vi "Voltage - Continuous Output.vi"(0 "Physical Channel(s)":tag="Dev1/ao0", 1 "Output Array":T2(array[cluster])=[{"Waveform Type"=0, "Amplitude"=1.0, "Frequency"=10.0}] {"Frequency" format="%0.2p"; "Amplitude" format="%0.2p"; "Waveform Type" items=["Sine Wave", "Triangle Wave", "Square Wave", "Sawtooth Wave"]}, 4 "Sample Rate":dbl=100000.0, 5 "Stop":bool, 7 "error in":errorcluster) -> (20 "Waveform Graph":waveform(dbl)[](graph)=[{"t0"=timestamp(0 s since 1904-01-01), "dt"=0.001, "Y"=[]}], 27 "error out":errorcluster)   [LabVIEW 2020]
uses:
  <vilib>/Utility/error.llb/DialogType.ctl
  <vilib>/DAQmx/write.llb/DAQmx Write (Analog 1D Wfm NChan NSamp).vi
  <vilib>/DAQmx/create/channels.llb/DAQmx Create Channel (AO-Voltage-Basic).vi
  <vilib>/DAQmx/configure/timing.llb/DAQmx Timing (Sample Clock).vi
  <vilib>/DAQmx/configure/trigger.llb/DAQmx Start Trigger (Digital Edge).vi
  <vilib>/DAQmx/configure/trigger.llb/DAQmx Start Trigger (Time).vi
  <vilib>/DAQmx/configure/trigger.llb/DAQmx Start Trigger (Analog Edge).vi
  <vilib>/DAQmx/miscellaneous.llb/DAQmx Fill In Error Info.vi
  <resource>/objmgr/daqmx.rc
  <vilib>/measure/NI_MABase.lvlib
panel:
  in  "Trigger Type":T1(tab)
  in  "Digital Start Trigger Edge":i32(ring)=10280 caption="Edge" items=["Rising"=10280, "Falling"=10171]
  in  "Digital Start Trigger Source":tag="/Dev1/PFI0" caption="Source"
  in  "Digital Pause Trigger Pause When":i32(ring)=10192 caption="Pause When" items=["High"=10192, "Low"=10214]
  in  "Digital Pause Trigger Source":tag="/Dev1/PFI0" caption="Source"
  in  "Analog Start Trigger Level":dbl caption="Level" format="%0.2f"
  in  "Analog Start Trigger Hysteresis":dbl caption="Hysteresis" format="%.2f"
  in  "Analog Start Trigger Slope":i32(ring)=10280 caption="Slope" items=["Rising"=10280, "Falling"=10171]
  in  "Analog Start Trigger Source":string="APFI0" caption="Source"
  in  "Analog Pause Trigger Source":string="APFI0" caption="Source"
  in  "Analog Pause Trigger Pause When":i32(ring)=10093 caption="Pause When" items=["Above Level"=10093, "Below Level"=10107]
  in  "Analog Pause Trigger Level":dbl caption="Level" format="%.2f"
  in  "When":timestamp
  in  "Select Time\nManually":bool
  in  "Number of Samples":i32=10000
  in  "Sample Clock Source":tag="OnboardClock"
  in  "Max Voltage":dbl=5.0
  in  "Min Voltage":dbl=-5.0
  out "Actual Sample Rate":dbl=1000.0 format="%0.2f"
  # "Channel Settings"
  # "Output"
  # "Timing and\nBuffer Settings"
  # "Waveform Settings"
  # "Trigger Settings"
  # "The number of elements in the waveform array must equal the number of channels in the task."
  # "To enable triggers, select a tab above, and configure the settings.\n\nNot all hardware supports all trigger types. Refer to your device documentation for more information."
  # "This trigger type is not supported in output tasks. \n\nRefer to your device documentation for more information on which triggers are supported."
  # "This trigger type is not supported in output tasks. \n\nRefer to your device documentation for more information on which triggers are supported."
  # "If time is not manually set, task will begin after 10 seconds"
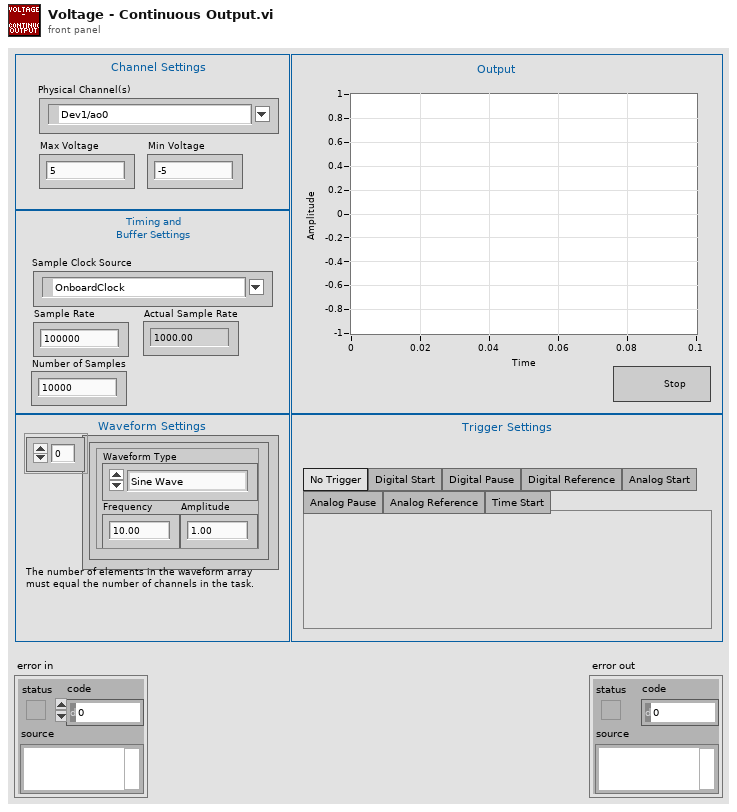
[diagram p1: front panel]
types:
  T1 = enum32{"No Trigger", "Digital Start", "Digital Pause", "Digital Reference", "Analog Start", "Analog Pause", "Analog Reference", "Time Start"}
  T2 = cluster{"Waveform Type":u16, "Amplitude":dbl, "Frequency":dbl}[]
  T3 = typedef "DialogType.ctl" = u16
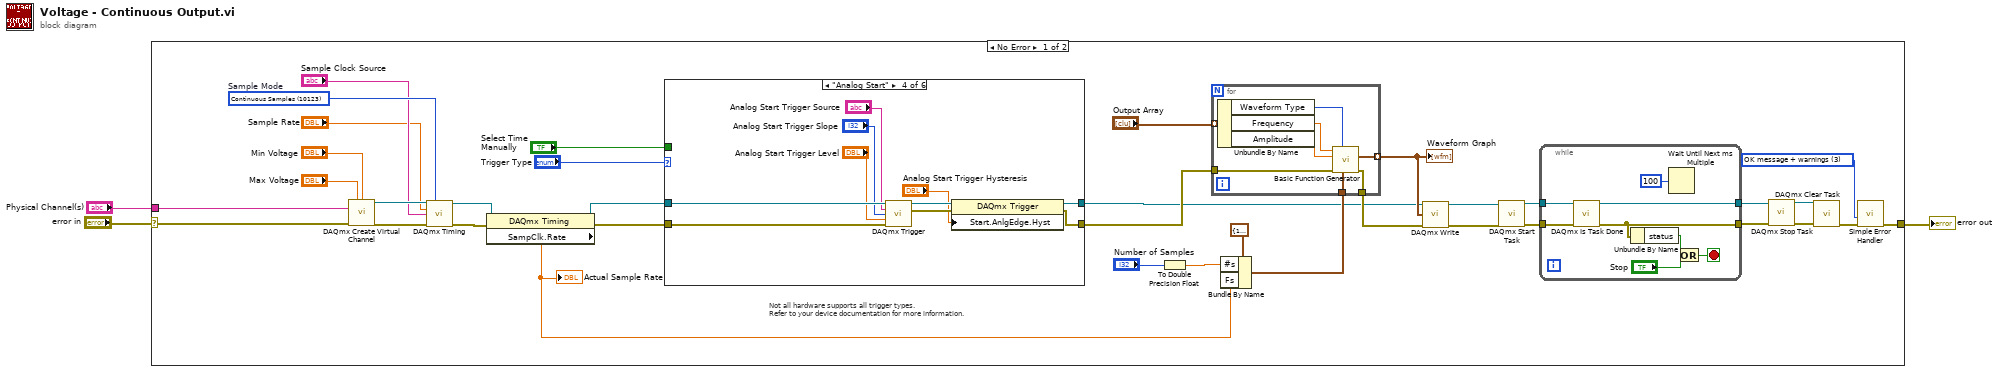
[diagram p0: block diagram]
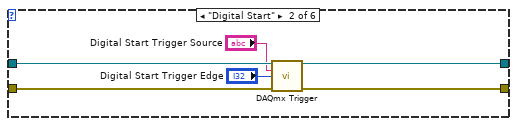
[diagram p3: hidden frame]
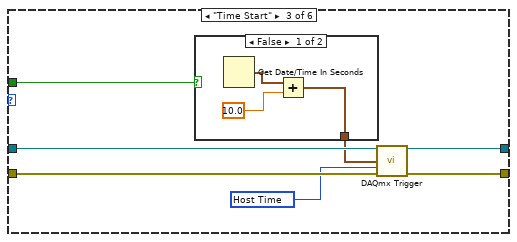
[diagram p4: hidden frame]
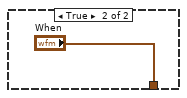
[diagram p5: hidden frame]
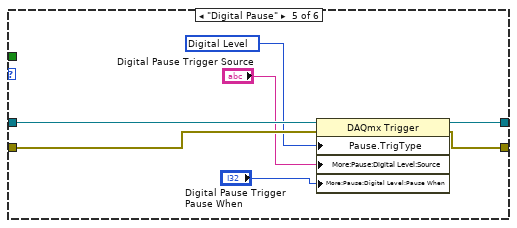
[diagram p6: hidden frame]
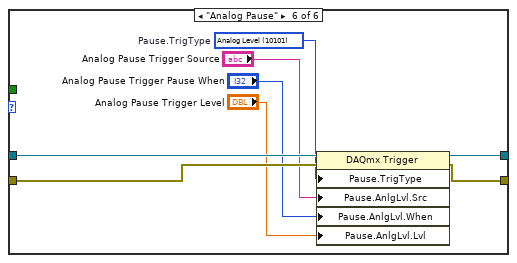
[diagram p7: hidden frame]
diagram:
  n1 = case shown="No Error" "error in" {
    selector: "error in" -> [w5 w100]
    tunnel: [w7 w100] -> w3
    tunnel: "Physical Channel(s)" -> [w6 _]
    frame No Error {
      w13 = T3 3 items=["no dialog", "OK message", "continue or stop message", "OK message + warnings", "continue/stop + warnings"] ("type of dialog (OK msg:1)")
      w37 = 10123 items=["Finite Samples"=10178, "Continuous Samples"=10123, "Hardware Timed Single Point"=12522]  # Sample Mode
      # "Not all hardware supports all trigger types.\nRefer to your device documentation for more information."
      n2 = call-poly <vilib>:"DAQmx Create Virtual Channel.vi"("maximum value"="Max Voltage", "minimum value"="Min Voltage", "physical channels"=w6, "error in"=w5) -> ("task out"=w35:refnum<k21>, "error out"=w36:errorcluster)  [unwired: 10 in]
      n3 = call-poly <vilib>:"DAQmx Timing.vi"("task/channels in"=w35, "sample mode"=w37, "rate"="Sample Rate", "source"="Sample Clock Source", "error in"=w36) -> ("task out"=w39:refnum<k21>, "error out"=w38:errorcluster)  [unwired: 9 in]
      n4 = property class="DAQmx Timing"(reference=w39, error in=w38) -> (reference out=w11:refnum<k21>, error out=w10:errorcluster, "SampClk.Rate"=w26:dbl)
      "Actual Sample Rate" <- w26
      n5 = case shown="\"Analog Start\"" "Trigger Type" {
        tunnel: w11 -> [w41 w47 w54 w68 w75 w83]
        tunnel: w10 -> [w40 w46 w53 w67 w72 w80]
        tunnel: [w41 w45 w52 w65 w74 w82] -> w8
        tunnel: [w40 w44 w51 w64 w73 w81] -> w9
        tunnel: "Select Time\nManually" -> [_ _ w48 _ _ _]
        frame "No Trigger", Default {
        }
        frame "Digital Start" {
          n6 = call-poly <vilib>:"DAQmx Trigger.vi"("task/channels in"=w47, "source"="Digital Start Trigger Source", "edge"="Digital Start Trigger Edge", "error in"=w46) -> ("task out"=w45:refnum<k21>, "error out"=w44:errorcluster)  [unwired: 10 in]
        }
        frame "Time Start" {
          w50 = 16126 items=["Host Time"=16126, "I/O Device Time"=16127] ("timescale")
          n7 = case shown="False" w48 {
            tunnel: [w56 "When"] -> w49
            frame False {
              n8 = Get Date/Time In Seconds() -> (seconds since 1Jan1904=w57:timestamp)
              n9 = Add(x=w57, y=10.0) -> (x+y=w56:timestamp)
            }
            frame True {
            }
          }
          n10 = call-poly <vilib>:"DAQmx Trigger.vi"("task/channels in"=w54, "when"=w49, "timescale"=w50, "error in"=w53) -> ("task out"=w52:refnum<k21>, "error out"=w51:errorcluster)  [unwired: 10 in]
        }
        frame "Analog Start" {
          n11 = call-poly <vilib>:"DAQmx Trigger.vi"("task/channels in"=w68, "source"="Analog Start Trigger Source", "slope"="Analog Start Trigger Slope", "level"="Analog Start Trigger Level", "error in"=w67) -> ("task out"=w63:refnum<k21>, "error out"=w62:errorcluster)  [unwired: 9 in]
          n12 = property class="DAQmx Trigger"(reference=w63, error in=w62, "Start.AnlgEdge.Hyst"="Analog Start Trigger Hysteresis") -> (reference out=w65:refnum<k21>, error out=w64:errorcluster)
        }
        frame "Digital Pause" {
          w71 = 10152 items=["Analog Level"=10101, "Analog Window"=10103, "Digital Level"=10152, "Digital Pattern"=10398, "None"=10230] ("Pause.TrigType")
          n13 = property class="DAQmx Trigger"(reference=w75, error in=w72, "Pause.TrigType"=w71, "More:Pause:Digital Level:Source"="Digital Pause Trigger Source", "More:Pause:Digital Level:Pause When"="Digital Pause Trigger Pause When") -> (reference out=w74:refnum<k21>, error out=w73:errorcluster)
        }
        frame "Analog Pause" {
          w79 = 10101 items=["Analog Level"=10101, "Analog Window"=10103, "Digital Level"=10152, "Digital Pattern"=10398, "None"=10230]  # Pause.TrigType
          n14 = property class="DAQmx Trigger"(reference=w83, error in=w80, "Pause.TrigType"=w79, "Pause.AnlgLvl.Src"="Analog Pause Trigger Source", "Pause.AnlgLvl.When"="Analog Pause Trigger Pause When", "Pause.AnlgLvl.Lvl"="Analog Pause Trigger Level") -> (reference out=w82:refnum<k21>, error out=w81:errorcluster)
        }
      }
      n15 = To Double Precision Float(number="Number of Samples") -> (double precision float=w19:dbl)
      n16 = Bundle By Name(cluster=cluster{"Fs":dbl, "#s":dbl} {"Fs"=1000.0, "#s"=1000.0} ("sampling info"), "#s"=w19, "Fs"=w26) -> (w25:cluster{"Fs":dbl, "#s":dbl})
      n17 = for {
        tunnel: w9 -> [w91]
        tunnel: w25 -> [w90]
        tunnel: [w89] -> w22
        tunnel: "Output Array" -> [w88] mode=indexing
        tunnel: [w84] -> w20 mode=indexing
        n18 = Unbundle By Name(w88) -> ("Waveform Type"=w87:u16, "Frequency"=w86:dbl, "Amplitude"=w85:dbl)
        n19 = call <vilib>:"Basic Function Generator.vi"("sampling info"=w90, "signal type"=w87, "error in (no error)"=w91, "amplitude"=w85, "frequency"=w86) -> ("error out"=w89:errorcluster, "signal out"=w84:waveform(dbl))  [unwired: 4 in, 1 out]
      }
      "Waveform Graph" <- w20
      n20 = call-poly <vilib>:"DAQmx Write.vi"("task/channels in"=w8, "data"=w20, "error in"=w22) -> ("task out"=w24:refnum<k21>, "error out"=w23:errorcluster)  [unwired: 10 in, 1 out]
      n21 = call <vilib>:"DAQmx Start Task.vi"("task/channels in"=w24, "error in"=w23) -> ("task out"=w34:refnum<k21>, "error out"=w33:errorcluster)  [unwired: 12 in]
      n22 = while {
        tunnel: w34 -> [w99]
        tunnel: w33 -> [w98]
        tunnel: [w95] -> w14
        tunnel: [w96] -> w15
        stop <- w97 stop-if-true
        n23 = call <vilib>:"DAQmx Is Task Done.vi"("task/channels in"=w99, "error in"=w98) -> ("task out"=w96:refnum<k21>, "error out"=w95:errorcluster)  [unwired: 11 in, 1 out]
        n24 = Unbundle By Name(w95) -> ("status"=w94:bool)
        n25 = Wait Until Next ms Multiple(millisecond multiple=u32 100) -> ()  [unwired: 1 out]
        n26 = Or(x=w94, y="Stop") -> (x .or. y?=w97:bool)
      }
      n27 = call <vilib>:"DAQmx Stop Task.vi"("task/channels in"=w15, "error in"=w14) -> ("task out"=w17:refnum<k21>, "error out"=w16:errorcluster)  [unwired: 12 in]
      n28 = call <vilib>:"DAQmx Clear Task.vi"("task in"=w17, "error in"=w16) -> ("error out"=w32:errorcluster)  [unwired: 13 in]
      n29 = call <vilib>:"Simple Error Handler.vi"("type of dialog (OK msg:1)"=w13, "error in (no error)"=w32) -> ("error out"=w7:errorcluster)  [unwired: 3 in, 4 out]
    }
    frame Error {
    }
  }
  "error out" <- w3
